vi "GetItfClassCluster.vi"(8 "error in (no error)":errorcluster, 10 "Interface Class":T1={"Experiment.lvclass"=refnum, "DataFileName"=path "", "HdrFileName"=path "", "DataFileRef"=refnum, "ScanParams"={"Entête"="", "Scan list"=[], "NbCourbe"=1, "IndCourbe"=0, "NomDon"=["RTêta;", "X&Y;"], "Session "=0, "Date"="", "Time"="", "VarParams"=[], "UserName"="", "ScanTableSize"=[], "VarPar list"=[], "DescKeyword"=""}, "DataQRefs"=[], "XYGraphCurves"=[], "AllCurves"=[], "CurvesParams"=[], "ScanGphInd"=[], "CurvesSetup"=[], "ScanDataQ"=[], "GraphRefArr"=[], "Graph_FA"=[], "FirstFreeFA"=0, "GraphConfig"=0, "PanRef"=refnum, "FAGraphNumArr"=[], "BaseDataPath"=path "", "ListBoxRef"=refnum, "VarParCount"=0, "GraphQRefArr"=[], "XScalesNames"=[], "YScalesNames"=[], "MainGraphQ"=refnum, "GraphEvent"=refnum, "2DGraphQRefArr"=[], "Scan2DGphInd"=[], "2DGraphRefArr"=[], "2DGphParams"=[], "GraphNumbers"=[], "LastGrphNum"=0, "AllDataQ"=[], "AllQRefs"=[], "VarParQRefs"=[], "DatQIndex"=[], "CalcQIndex"=[], "SubVarParQRefs"=[], "AllVarParQ"=[], "UseSubFolder"=FALSE}, 11 "Interface.lvclass":refnum<class "Interface.lvclass">) -> (0 "error out":errorcluster, 3 "Interface.lvclass Out":refnum<class "Interface.lvclass">)   [LabVIEW 2019, in "Interface.lvclass"]
uses:
  Interface.lvclass
  ItfDataCluster.ctl
  Experiment Class/Experiment.lvclass
  ScanParams.ctl
  CurveSetup.ctl
  2DGraphSetup.ctl
  Interface.lvclass/Interface.ctl
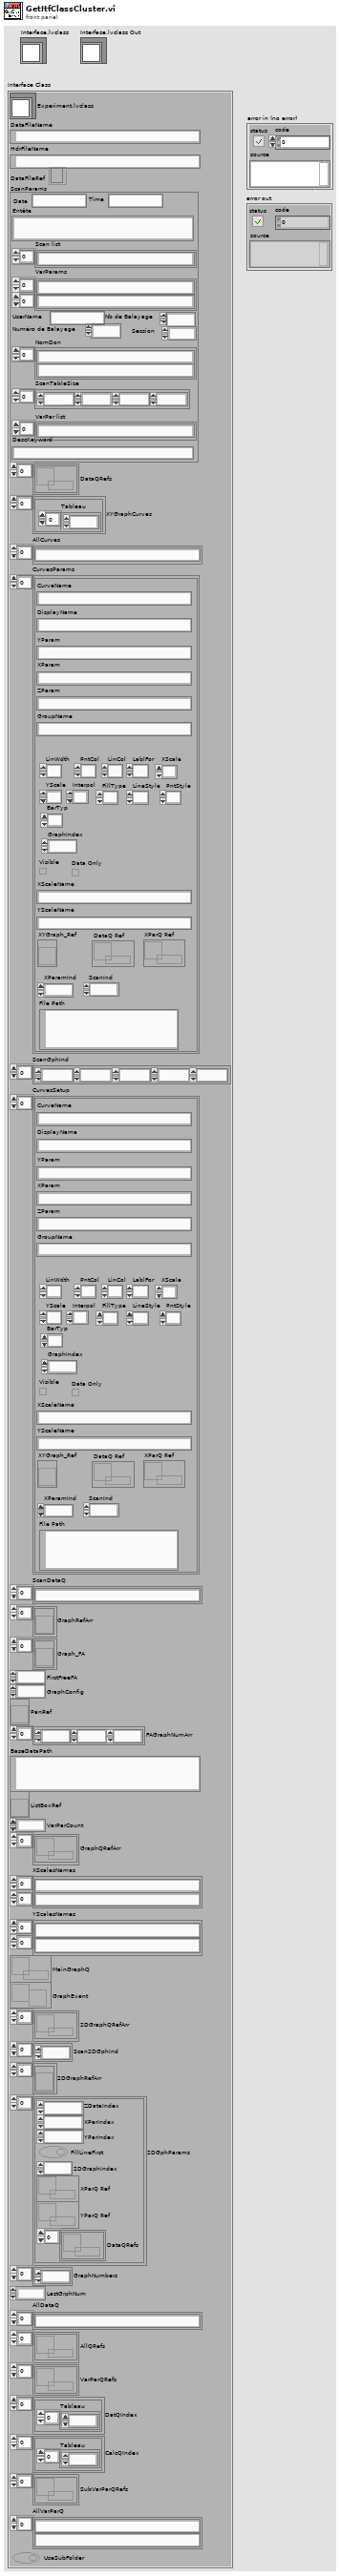
[diagram p1: front panel]
types:
  T1 = typedef "ItfDataCluster.ctl" = cluster{"Experiment.lvclass":refnum<class "Experiment.lvclass">, "DataFileName":path, "HdrFileName":path, "DataFileRef":refnum<file>, "ScanParams":T2, "DataQRefs":refnum<queue>[], "XYGraphCurves":cluster{"Tableau":i32[]}[], "AllCurves":string[], "CurvesParams":T3[], "ScanGphInd":i32[], "CurvesSetup":T3[], "ScanDataQ":string[], "GraphRefArr":refnum<vi>[], "Graph_FA":refnum<vi>[], "FirstFreeFA":u8, "GraphConfig":i32, "PanRef":refnum<vi>, "FAGraphNumArr":i32[], "BaseDataPath":path, "ListBoxRef":refnum<vi>, "VarParCount":i32, "GraphQRefArr":refnum<queue>[], "XScalesNames":string[][], "YScalesNames":string[][], "MainGraphQ":refnum<queue>, "GraphEvent":refnum<user-event>, "2DGraphQRefArr":refnum<queue>[], "Scan2DGphInd":i32[], "2DGraphRefArr":refnum<vi>[], "2DGphParams":T4[], "GraphNumbers":i32[], "LastGrphNum":i32, "AllDataQ":string[], "AllQRefs":refnum<queue>[], "VarParQRefs":refnum<queue>[], "DatQIndex":cluster{"Tableau":i32[]}[], "CalcQIndex":cluster{"Tableau":i32[]}[], "SubVarParQRefs":refnum<queue>[], "AllVarParQ":string[], "UseSubFolder":bool}
  T2 = typedef "Interface.lvclass/ScanParams.ctl" = cluster{"Entête":string, "Scan list":string[], "NbCourbe":i32, "IndCourbe":i64, "NomDon":string[], "Session ":i32, "Date":string, "Time":string, "VarParams":string[][], "UserName":string, "ScanTableSize":i32[], "VarPar list":string[], "DescKeyword":string}
  T3 = typedef "Interface.lvclass/CurveSetup.ctl" = cluster{"CurveName":string, "YParam":string, "XParam":string, "ZParam ":string, "GroupName":string, "LinWdth":u8, "PntCol":u32, "LinCol":u32, "LablFor":u8, "XScale":u32, "YScale":u32, "Interpol":u8, "DisplayName":string, "FillType":i16, "LineStyle":u8, "PntStyle":u8, "BarTyp":u8, "GraphIndex":i32, "Visible":bool, "XScaleName":string, "YScaleName":string, "XYGraph_Ref":refnum<vi>, "Data Only":bool, "DataQ Ref":refnum<queue>, "XParQ Ref":refnum<queue>, "XParamInd":i32, "ScanInd":i32, "File Path":path}
  T4 = typedef "2DGraphSetup.ctl" = cluster{"ZDataIndex":i32, "XParIndex":i32, "YParIndex":i32, "FillLineFirst":bool, "2DGraphIndex":i32, "XParQ Ref":refnum<queue>, "YParQ Ref":refnum<queue>, "DataQRefs":refnum<queue>[]}
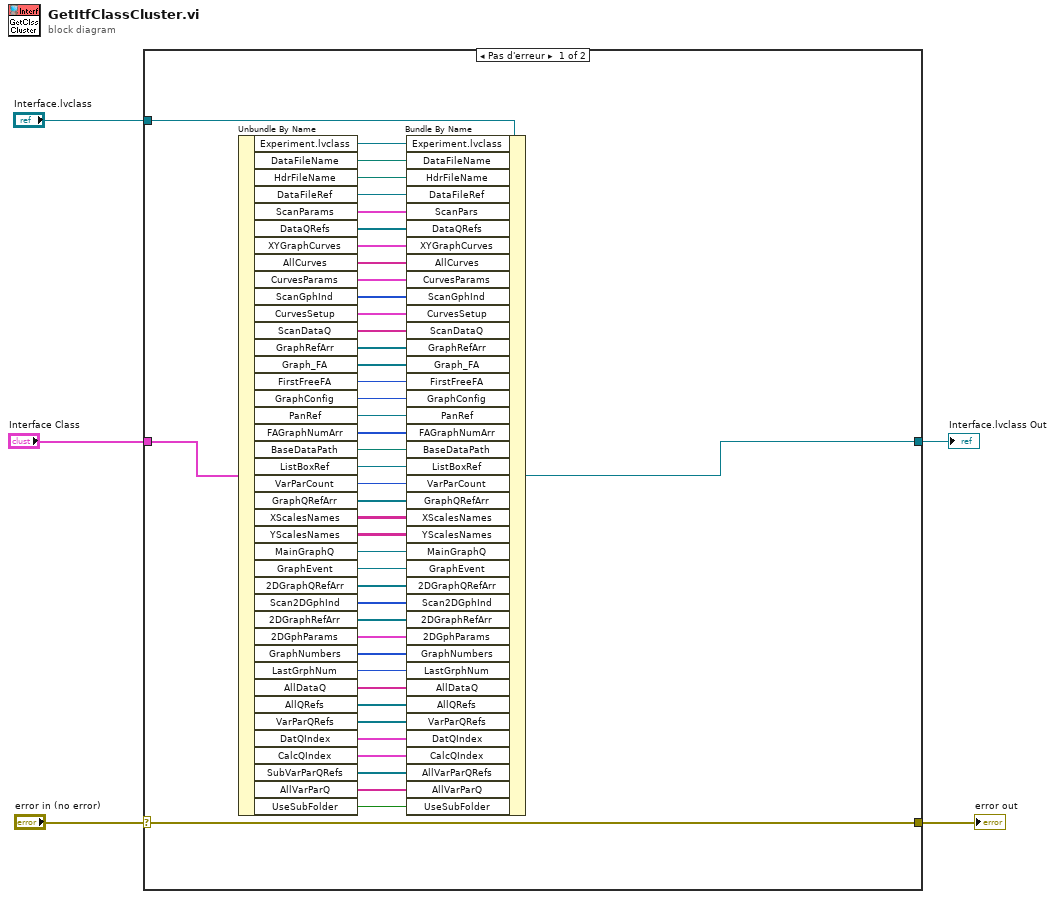
[diagram p0: block diagram]
diagram:
  n1 = case shown="Pas d'erreur" "error in (no error)" {
    selector: "error in (no error)" -> [w15 w51]
    tunnel: [w15 w51] -> w4
    tunnel: [w12 w50] -> w3
    tunnel: "Interface.lvclass" -> [w13 w50]
    tunnel: "Interface Class" -> [w14 _]
    frame No Error {
      n2 = Unbundle By Name(w14) -> ("Experiment.lvclass"=w49:refnum<class "Experiment.lvclass">, "DataFileName"=w48:path, "HdrFileName"=w47:path, "DataFileRef"=w46:refnum<file>, "ScanParams"=w45:T2, "DataQRefs"=w44:refnum<queue>[], "XYGraphCurves"=w43:cluster{"Tableau":i32[]}[], "AllCurves"=w42:string[], "CurvesParams"=w41:T3[], "ScanGphInd"=w40:i32[], "CurvesSetup"=w39:T3[], "ScanDataQ"=w38:string[], "GraphRefArr"=w37:refnum<vi>[], "Graph_FA"=w36:refnum<vi>[], "FirstFreeFA"=w35:u8, "GraphConfig"=w34:i32, "PanRef"=w33:refnum<vi>, "FAGraphNumArr"=w32:i32[], "BaseDataPath"=w31:path, "ListBoxRef"=w30:refnum<vi>, "VarParCount"=w29:i32, "GraphQRefArr"=w28:refnum<queue>[], "XScalesNames"=w27:string[][], "YScalesNames"=w26:string[][], "MainGraphQ"=w25:refnum<queue>, "GraphEvent"=w24:refnum<user-event>, "2DGraphQRefArr"=w23:refnum<queue>[], "Scan2DGphInd"=w22:i32[], "2DGraphRefArr"=w21:refnum<vi>[], "2DGphParams"=w20:T4[], "GraphNumbers"=w19:i32[], "LastGrphNum"=w18:i32, "AllDataQ"=w17:string[], "AllQRefs"=w16:refnum<queue>[], "VarParQRefs"=w11:refnum<queue>[], "DatQIndex"=w10:cluster{"Tableau":i32[]}[], "CalcQIndex"=w9:cluster{"Tableau":i32[]}[], "SubVarParQRefs"=w8:refnum<queue>[], "AllVarParQ"=w7:string[], "UseSubFolder"=w6:bool)
      n3 = Bundle By Name(cluster=w13, "Experiment.lvclass"=w49, "DataFileName"=w48, "HdrFileName"=w47, "DataFileRef"=w46, "ScanPars"=w45, "DataQRefs"=w44, "XYGraphCurves"=w43, "AllCurves"=w42, "CurvesParams"=w41, "ScanGphInd"=w40, "CurvesSetup"=w39, "ScanDataQ"=w38, "GraphRefArr"=w37, "Graph_FA"=w36, "FirstFreeFA"=w35, "GraphConfig"=w34, "PanRef"=w33, "FAGraphNumArr"=w32, "BaseDataPath"=w31, "ListBoxRef"=w30, "VarParCount"=w29, "GraphQRefArr"=w28, "XScalesNames"=w27, "YScalesNames"=w26, "MainGraphQ"=w25, "GraphEvent"=w24, "2DGraphQRefArr"=w23, "Scan2DGphInd"=w22, "2DGraphRefArr"=w21, "2DGphParams"=w20, "GraphNumbers"=w19, "LastGrphNum"=w18, "AllDataQ"=w17, "AllQRefs"=w16, "VarParQRefs"=w11, "DatQIndex"=w10, "CalcQIndex"=w9, "AllVarParQRefs"=w8, "AllVarParQ"=w7, "UseSubFolder"=w6) -> (w12:refnum<class "Interface.lvclass">)
    }
    frame Error {
    }
  }
  "error out" <- w4
  "Interface.lvclass Out" <- w3
